vi "Test_2D_array_index_speed.vi"() -> ()   [LabVIEW 2018]
panel:
  out "per replacement, us":dbl
  out "Output":i32[][](array[numeric])
  in  "Array size (side)":i32=1000
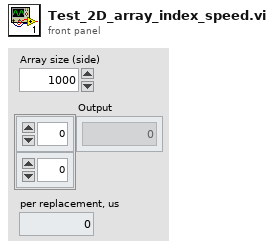
[diagram p1: front panel]
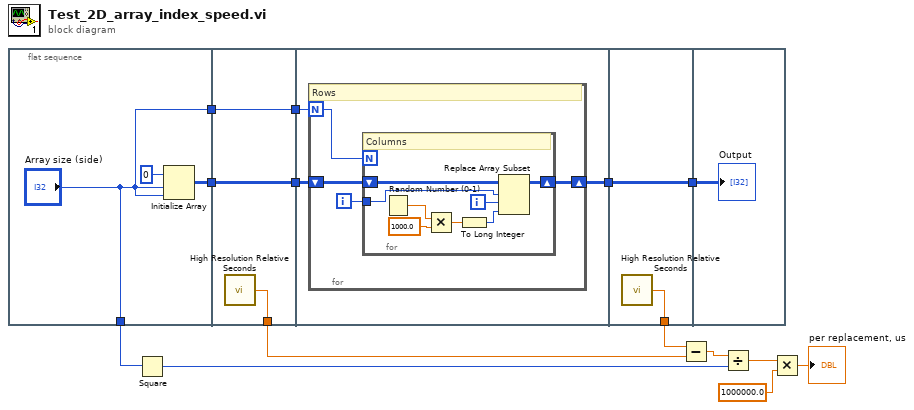
[diagram p0: block diagram]
diagram:
  n1 = flat-sequence {
    tunnel: [w16] -> w13
    tunnel: ["Array size (side)"] -> w11
    tunnel: ["Array size (side)"] -> w5
    tunnel: [w20] -> w14
    tunnel: w13 -> [w20]
    tunnel: [w19] -> w12
    tunnel: w11 -> [w19]
    tunnel: [w18] -> w7
    tunnel: w14 -> [w23]
    tunnel: w12 -> [w22]
    tunnel: [w21] -> w9
    tunnel: [w37] -> w10
    tunnel: w9 -> [w37]
    tunnel: [w36] -> w8
    tunnel: w10 -> [w38]
    frame #0 {
      n2 = Initialize Array(0, "Array size (side)", "Array size (side)") -> (w16:i32[][])
    }
    frame #1 {
      n3 = call <vilib>:"High Resolution Relative Seconds.vi"() -> ("relative seconds"=w18:dbl)
    }
    frame #2 {
      n4 = for {
        N: w22 -> [w24]
        shift-right: [w26] -> w21
        shift-left: w23 -> [w27]
        i -> [w25]
        # "Rows"
        n5 = for {
          N: w24 -> [_]
          shift-right: [w31] -> w26
          shift-left: w27 -> [w32]
          tunnel: w25 -> [w29]
          i -> [w28]
          # "Columns"
          n6 = Random Number (0-1)() -> (number: 0 to 1=w35:dbl)
          n7 = Multiply(x=w35, y=1000.0) -> (x*y=w33:dbl)
          n8 = To Long Integer(number=w33) -> (32bit integer=w30:i32)
          n9 = Replace Array Subset(array=w32, new element=w30, index (row)=w29, index (col)=w28) -> (w31:i32[][])
        }
      }
    }
    frame #3 {
      n10 = call <vilib>:"High Resolution Relative Seconds.vi"() -> ("relative seconds"=w36:dbl)
    }
    frame #4 {
      "Output" <- w38
    }
  }
  n11 = Square(x=w5) -> (x^2=w4:i32)
  n12 = Subtract(x=w8, y=w7) -> (x-y=w6:dbl)
  n13 = Divide(x=w6, y=w4) -> (x/y=w3:dbl)
  n14 = Multiply(x=w3, y=1000000.0) -> (x*y=→"per replacement, us":dbl)
